vi "Flock_Master_ReadCurRev.vi"(0 "configuration file path":path, 11 "error in (no error)":errorcluster) -> (3 "BranchNum":i32, 4 "MajorRev":i32, 6 "MinorRev":i32, 8 "BuildPhase":string, 10 "BuildNum":i32, 15 "error out":errorcluster)   [LabVIEW 2014, in "Flock_Master_BuildRevision.lvlib"]
uses:
  Flock_Master_BuildRevision.lvlib
  <vilib>/Utility/config.llb/Read Key (I32).vi
  <vilib>/Utility/config.llb/Read Key (String).vi
  <vilib>/Utility/config.llb/NI_LVConfig.lvlib
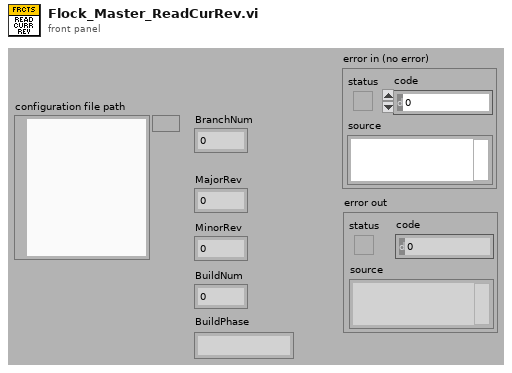
[diagram p1: front panel]
types:
  T1 = typedef "NI_LVConfig.lvlib/Config Data RefNum.ctl" = refnum<k1>
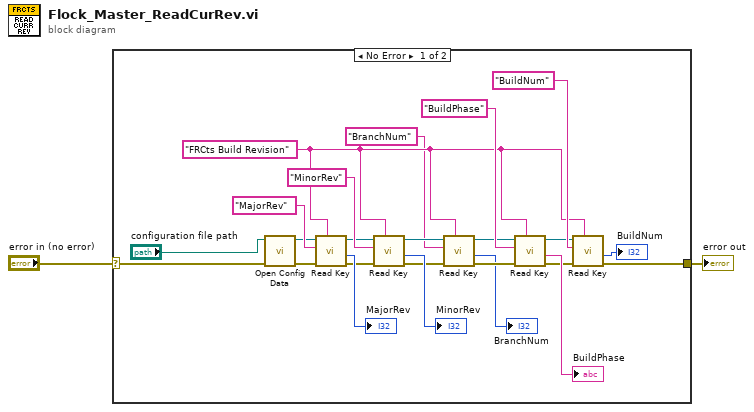
[diagram p0: block diagram]
diagram:
  n1 = case shown="No Error" "error in (no error)" {
    selector: "error in (no error)" -> [w10 w27]
    tunnel: [w11 w27] -> w2
    frame No Error {
      w7 = "FRCts Build Revision"
      n2 = call <vilib>:"Open Config Data.vi"("error in (no error)"=w10, "configuration file path"="configuration file path") -> ("error out"=w14:errorcluster, "refnum"=w13:T1)  [unwired: 7 in, 1 out]
      n3 = call-poly <vilib>:"Read Key.vi"("section"=w7, "error in (no error)"=w14, "key"="MajorRev", "refnum"=w13) -> ("error out"=w17:errorcluster, "value"=→"MajorRev":i32, "refnum out"=w16:T1)  [unwired: 4 in, 1 out]
      n4 = call-poly <vilib>:"Read Key.vi"("section"=w7, "error in (no error)"=w17, "key"="MinorRev", "refnum"=w16) -> ("error out"=w9:errorcluster, "value"=→"MinorRev":i32, "refnum out"=w8:T1)  [unwired: 4 in, 1 out]
      n5 = call-poly <vilib>:"Read Key.vi"("section"=w7, "error in (no error)"=w9, "key"="BranchNum", "refnum"=w8) -> ("error out"=w5:errorcluster, "value"=→"BranchNum":i32, "refnum out"=w4:T1)  [unwired: 4 in, 1 out]
      n6 = call-poly <vilib>:"Read Key.vi"("section"=w7, "error in (no error)"=w5, "key"="BuildPhase", "refnum"=w4) -> ("error out"=w20:errorcluster, "value"=→"BuildPhase":string, "refnum out"=w21:T1)  [unwired: 4 in, 1 out]
      n7 = call-poly <vilib>:"Read Key.vi"("section"=w7, "error in (no error)"=w20, "key"="BuildNum", "refnum"=w21) -> ("error out"=w11:errorcluster, "value"=→"BuildNum":i32)  [unwired: 4 in, 2 out]
    }
    frame Error {
    }
  }
  "error out" <- w2
